vi "Timestamp to Datetime String.vi"(1 "Timestamp":timestamp) -> (0 "Date-Time String":string)   [LabVIEW 2023, in "Error Manager.lvlib" / "Error Log.lvclass"]
uses:
  Error Log.lvclass
  Error Log.lvclass/Error Log.ctl
panel:
  # "Input\nInputs to the VI"
  # "Development\nControls or indicators that are useful for development or testing, but which are not outputs of the VI."
  # "Output\nOutputs of the VI"
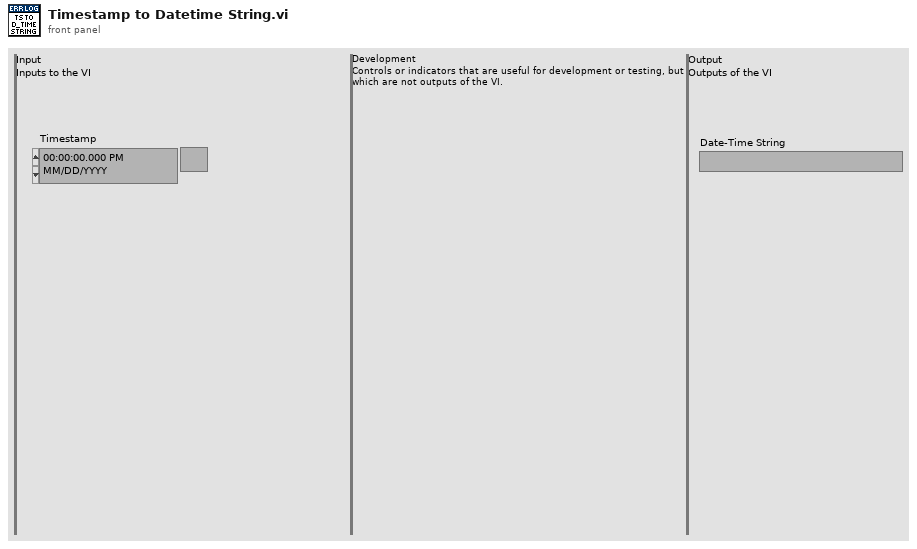
[diagram p1: front panel]
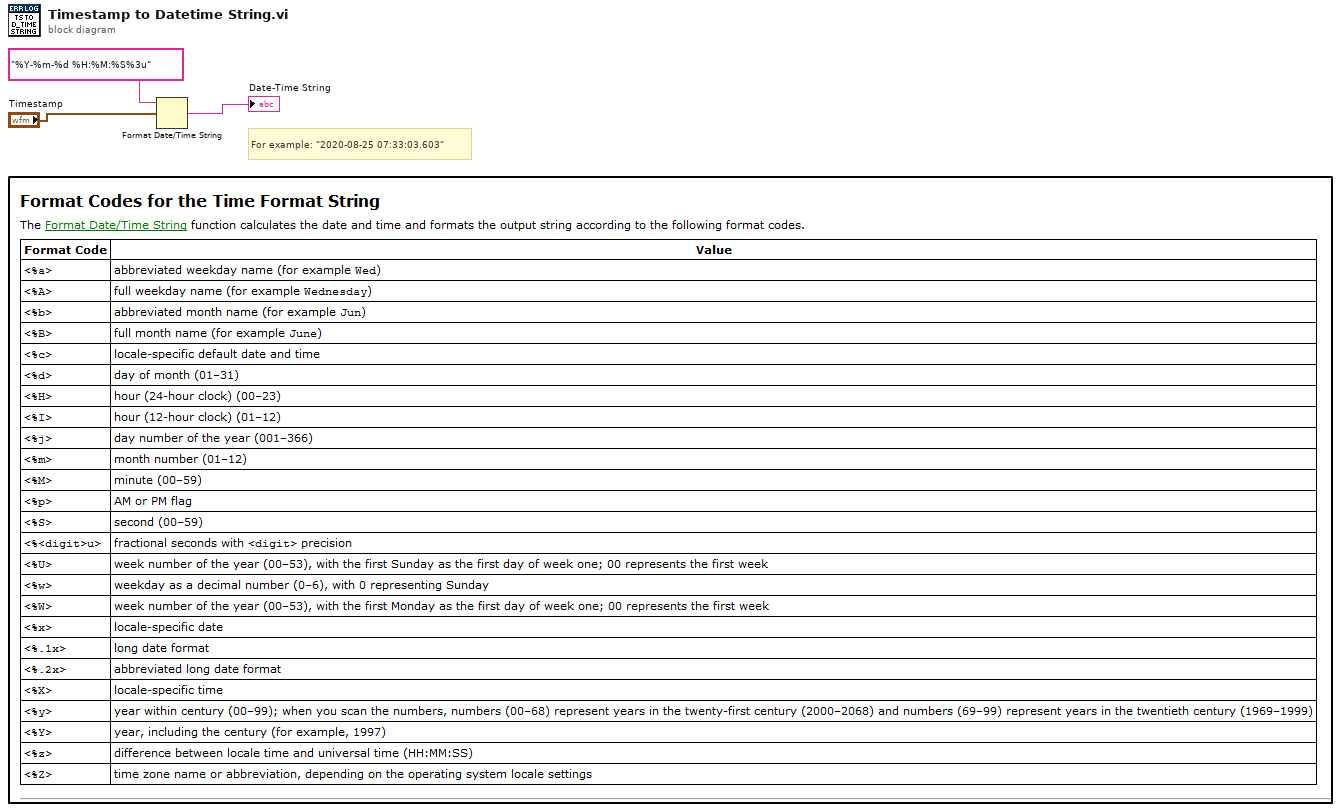
[diagram p0: block diagram]
diagram:
  # "For example: \"2020-08-25 07:33:03.603\""
  n1 = Format Date/Time String(time format string (%c)="%Y-%m-%d %H:%M:%S%3u", seconds (now)="Timestamp") -> (date/time string=→"Date-Time String":string)  [unwired: 1 in]
